vi "Autonics_1Scan_KAERI_lab2.vi"() -> ()   [LabVIEW 2018]
uses:
  <vilib>/Platform/NI_3dgraph.lvlib
  <vilib>/Utility/file.llb/Write To Spreadsheet File (DBL).vi
  <vilib>/Analysis/Matrix/Datatypes/RealMatrix.ctl
  <vilib>/Analysis/Matrix/NI_Matrix.lvlib
  <resource>/objmgr/daqmx.rc
  <vilib>/Instr/_visa.llb/VISA Configure Serial Port (Instr).vi
  <vilib>/DAQmx/configure/trigger.llb/DAQmx Start Trigger (Digital Edge).vi
  <vilib>/DAQmx/read.llb/DAQmx Read (Analog 2D DBL NChan NSamp).vi
  <vilib>/DAQmx/configure/timing.llb/DAQmx Timing (Sample Clock).vi
  <vilib>/DAQmx/create/channels.llb/DAQmx Create Channel (AI-Voltage-Basic).vi
  <vilib>/Analysis/NI_AALPro.lvlib
  <vilib>/Utility/file.llb/Read From Spreadsheet File (DBL).vi
  <vilib>/Analysis/2dsp.llb/Real FFT.vi
  <vilib>/Analysis/3filter.llb/Filter Passband Type.ctl
  <vilib>/Analysis/NI_AALBase.lvlib
panel:
  in  "Inverse":bool
  out "Sum Abs":dbl
  in  "Even":bool
  in  "Odd":bool
  in  "Scan Mode":bool
  in  "Save Analysis":bool caption="Save Process"
  in  "Open":bool
  in  "Filter?":bool
  in  "Direction":u16(ring) items=["X-dir", "Y-dir"]
  in  "filter type":T1
  in  "Sampling Hz":dbl=1000.0
  in  "High Cutoff Hz":dbl=300.0
  in  "Low Cutoff Hz":dbl=50.0
  in  "Order":dbl=2.0
  in  "Transpose ?":bool
  in  "3D Surface Analysis":refnum<k7>(container)
  in  "Color Min":dbl step=0.01
  in  "Color Max":dbl=1.0 step=0.01
  in  "Auto Scale ?":bool
  in  "Area View":bool
  out "Cursor X":dbl=1.0
  out "Cursor Y":dbl=1.0
  out "Cursor Z":dbl=1.0
  out "Section View Y":dbl[](graph) caption="Section View"
  in  "Line X":dbl
  in  "Line Y":dbl
  in  "Repair Line X":bool
  in  "Repair Line Y":bool
  in  "Back data Analysis":bool
  in  "dX":bool
  in  "dY":bool
  out "XY Graph":cluster{"Array Repaired":dbl[], dbl[]}(graph)
  in  "X-max":dbl
  in  "X-min":dbl
  in  "Trim Data":bool
  in  "Y-max":dbl
  in  "Y-min":dbl
  in  "ViewMode Analysis":i32(ring) items=["cwViewXYPlane", "cwViewXZPlane", "cwViewYZPlane", "cwViewUserDefined"]
  in  "Plot style Analysis":i32(ring)=5 items=["cwLine"=1, "cwPoint"=2, "cwLinePoint"=3, "cwHiddenLine"=4, "cwSurface"=5, "cwSurfaceLine"=6, "cwSurfaceNormal"=7, "cwContourLine"=8, "cwSurfaceContour"=9]
  out "Section View 2":dbl[](graph) caption="Section View"
  in  "Scan Distance":dbl=350.0
  in  "Multiplier":dbl=10.0
  in  "Save Button":bool caption="Save Process"
  in  "ViewMode":i32(ring) items=["cwViewXYPlane", "cwViewXZPlane", "cwViewYZPlane", "cwViewUserDefined"]
  in  "Back data":bool
  in  "Data Type":u16(ring) items=["Normal", "dX", "dY"]
  in  "Sampling Rate(Hz)":dbl=15000.0
  in  "Samples per Channels":i32=1000
  in  "Min Volts":dbl=-10.0 format="%0.2f"
  in  "Max Volts":dbl=10.0 format="%0.2f"
  in  "Channels":tag="Dev3/ai0:63"
  in  "Scan Step (mm)":dbl=1.0
  in  "Scan":bool
  in  "Plot style":i32(ring)=5 items=["cwLine"=1, "cwPoint"=2, "cwLinePoint"=3, "cwHiddenLine"=4, "cwSurface"=5, "cwSurfaceLine"=6, "cwSurfaceNormal"=7, "cwContourLine"=8, "cwSurfaceContour"=9]
  in  "3D Surface":refnum<k7>(container)
  in  "Flow control":u16(ring) items=["None", "XON/XOFF", "RTS/CTS", "XON/XOFF & RTS/CTS", "DTR/DSR", "XON/XOFF & DTR/DSR"]
  in  "Stop bits":u16(ring)=10 items=["1.0"=10, "1.5"=15, "2.0"=20]
  in  "Parity":dbl
  in  "Data bits":u16=8 min=5 max=8 step=1
  in  "Baud Rate":u32=57600
  in  "COM Port":refnum<visa-resource-name>="COM3"
  in  "Travel per Pulse (mm)":dbl=0.002
  in  "Speed (mm/s)":dbl=10.0
  out "Current  Position (mm)":dbl format="%#_4g"
  in  "Move Distance (mm)":dbl=20.0
  in  "Stop Scan":bool
  in  "Stop":bool
  in  "Home":bool
  in  "Right":bool
  in  "Left":bool
  # "SCANNER CONTROL"
  # "BOBBIN-TYPE MAGNETIC CAMERA"
  # "CHANNELS"
  # "COM Setting"
  # "TIMING"
  # "DATA ANALYSIS"
  # "Filters"
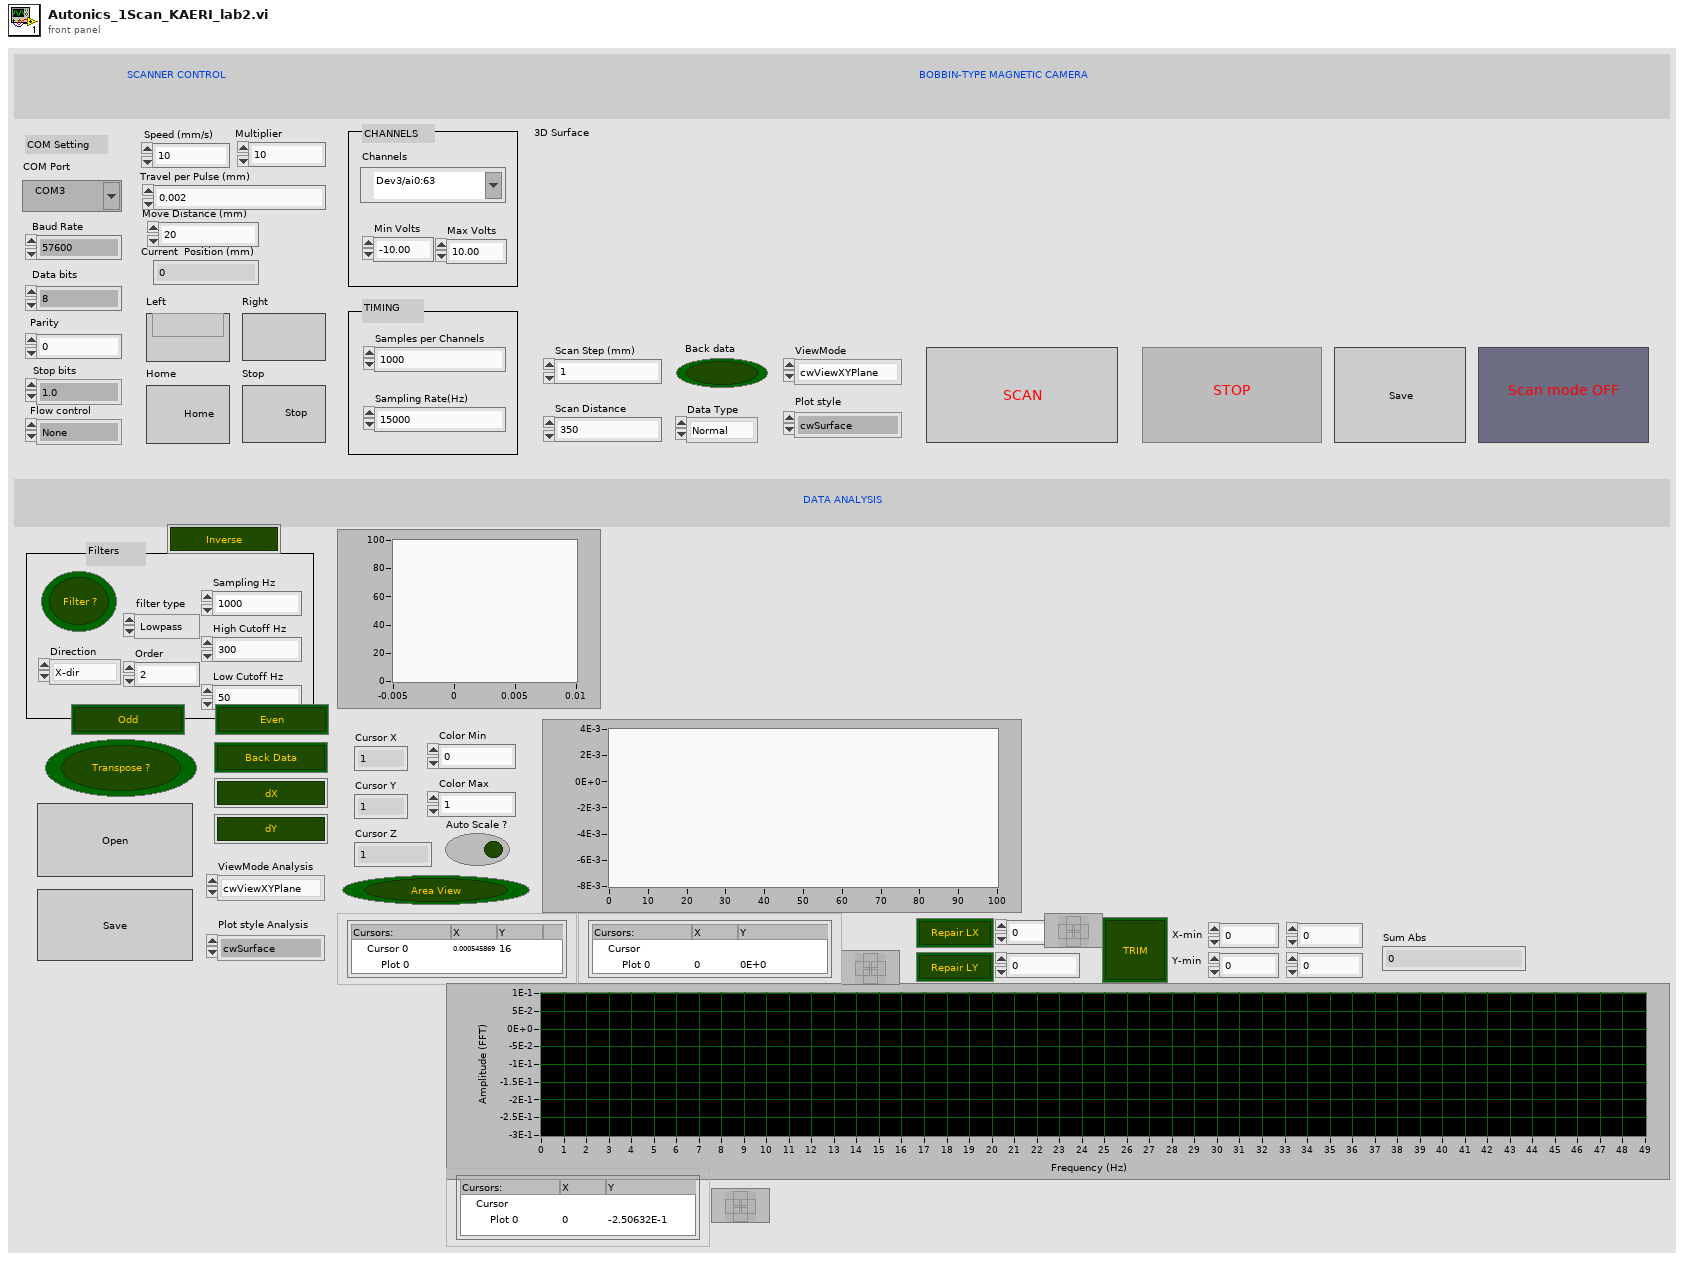
[diagram p1: front panel]
types:
  T1 = typedef "NI_AALBase.lvlib/Filter Passband Type.ctl" = enum32{"Lowpass", "Highpass", "Bandpass", "Bandstop"}
  T2 = typedef "NI_Matrix.lvlib/RealMatrix.ctl" = dbl[][]
  T3 = enum32{"Invalid", "Standard", "Closed", "Hidden", "Minimized", "Maximized"}
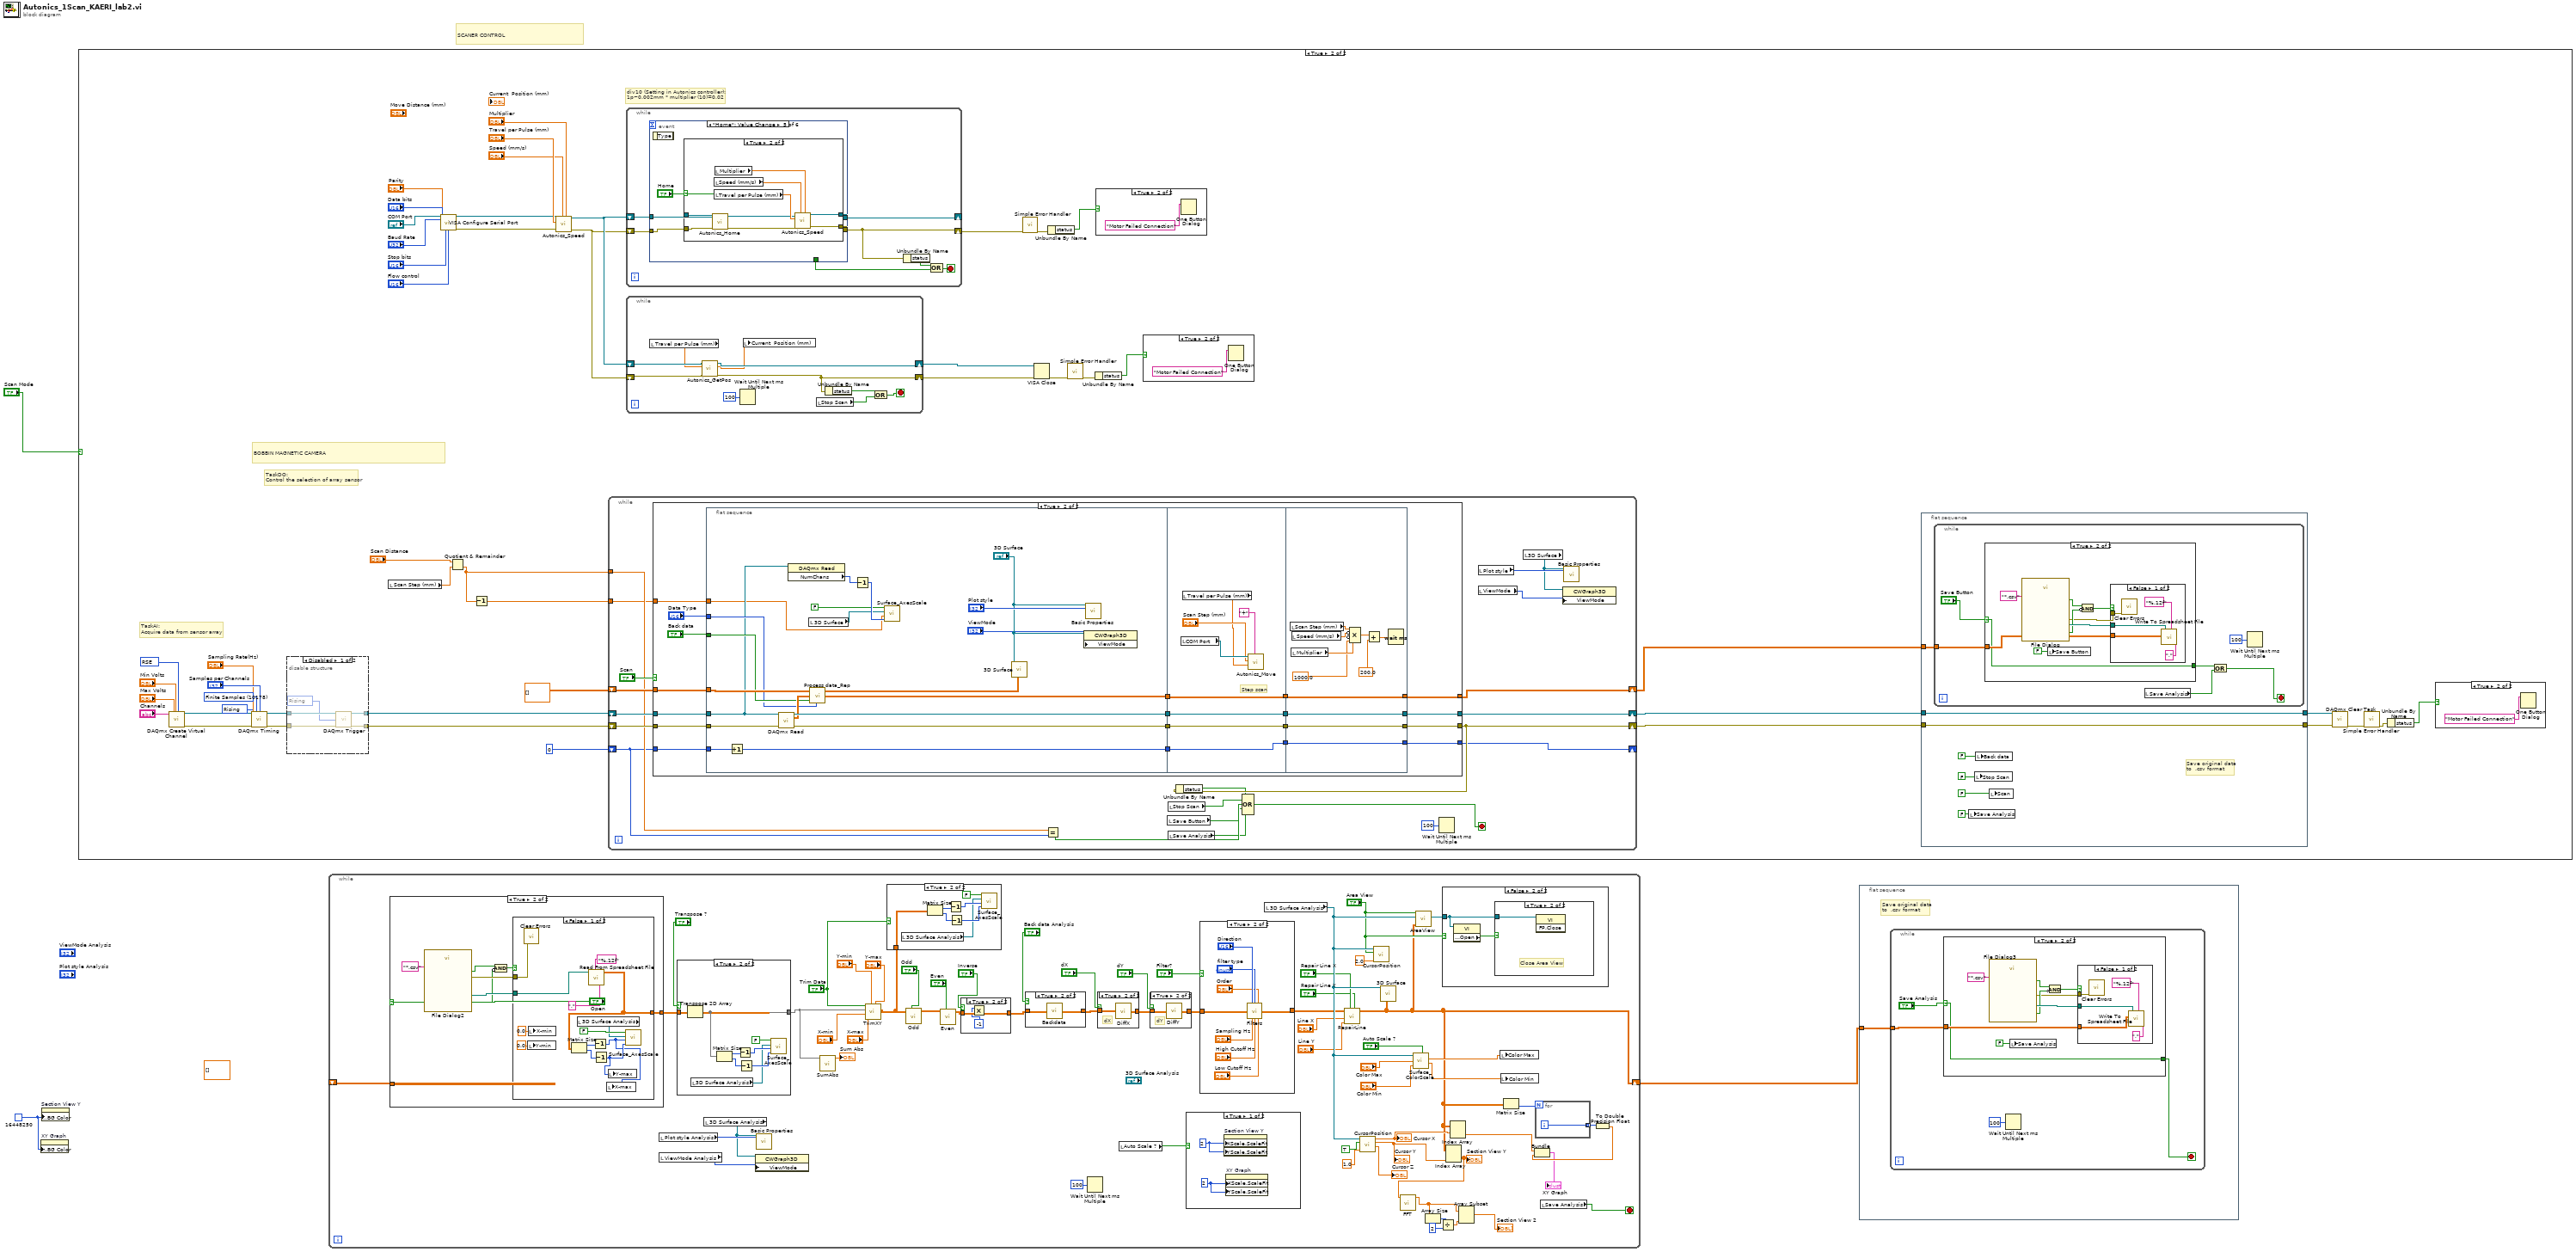
[diagram p0: block diagram]
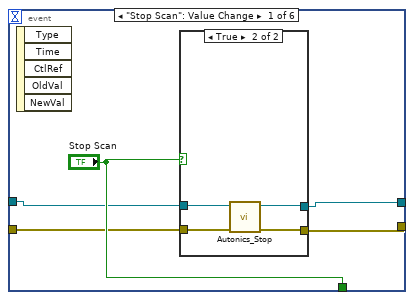
[diagram p5: hidden frame]
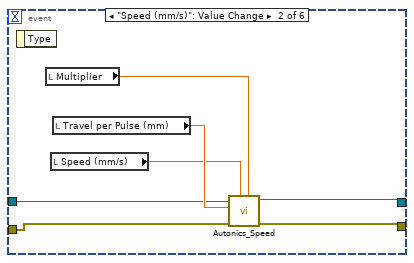
[diagram p7: hidden frame]
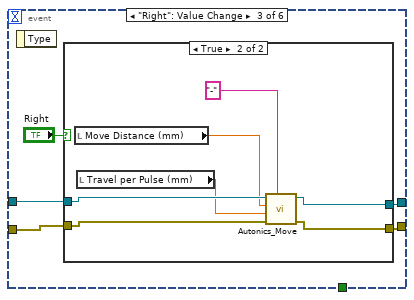
[diagram p8: hidden frame]
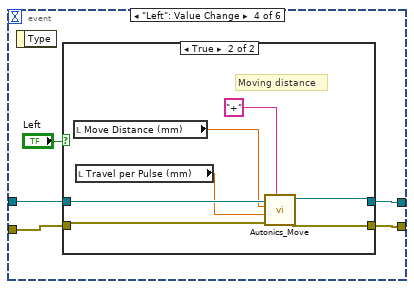
[diagram p10: hidden frame]
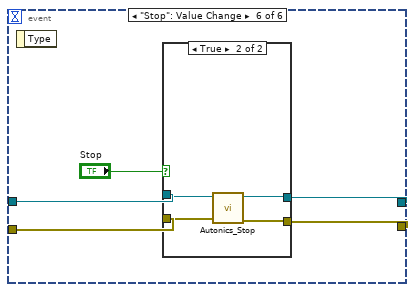
[diagram p13: hidden frame]
diagram:
  w2 = u32 16448250
  (unwired) T2 [] ("Output (Matrix)")
  # "SCANER CONTROL"
  n1 = property on="XY Graph" class="XYGraph (strict)"("Plot Area:Colors:BG Color"=w2) -> ()  [unwired: 2 in, 2 out]
  n2 = property on="Section View Y" class="WFGraph (strict)"("Plot Area:Colors:BG Color"=w2) -> ()  [unwired: 2 in, 2 out]
  n3 = case shown="True" "Scan Mode" {
    frame False {
    }
    frame True {
      w35 = 10280 items=["Rising"=10280, "Falling"=10171] ("active edge")
      w44 = 10083 items=["default"=-1, "RSE"=10083, "NRSE"=10078, "Differential"=10106, "Pseudodifferential"=12529] ("input terminal configuration")
      w45 = 10178 items=["Finite Samples"=10178, "Continuous Samples"=10123, "Hardware Timed Single Point"=12522] ("sample mode")
      # "div10 (Setting in Autonics controller):\n1p~0.002mm * multiplier (10)=0.02"
      # "TaskAI:\nAcquire data from sensor array"
      # "TaskDO: \nControl the selection of array sensor"
      # "BOBBIN MAGNETIC CAMERA"
      n4 = call-poly <vilib>:"DAQmx Create Virtual Channel.vi"("maximum value"="Max Volts", "minimum value"="Min Volts", "input terminal configuration"=w44, "physical channels"="Channels") -> ("task out"=w52:refnum<k21>, "error out"=w51:errorcluster)  [unwired: 10 in]
      n5 = call-poly <vilib>:"DAQmx Timing.vi"("task/channels in"=w52, "sample mode"=w45, "samples per channel"="Samples per Channels", "rate"="Sampling Rate(Hz)", "active edge"=w35, "error in"=w51) -> ("task out"=w34:refnum<k21>, "error out"=w33:errorcluster)  [unwired: 8 in]
      n6 = disable-structure shown="Disabled" {
        disable-tunnel: w34 -> [w151 w153]
        disable-tunnel: [w150 w153] -> w29
        disable-tunnel: w33 -> [w149 w152]
        disable-tunnel: [w148 w152] -> w32
        frame Disabled {
          w147 = 10280 items=["Rising"=10280, "Falling"=10171] ("edge")
          n7 = call-poly <vilib>:"DAQmx Trigger.vi"("task/channels in"=w151, "edge"=w147, "error in"=w149) -> ("task out"=w150:refnum<k21>, "source"=w146:tag, "error out"=w148:errorcluster)  [unwired: 10 in]
        }
        frame Enabled {
        }
      }
      n8 = local read "Scan Step (mm)"() -> (w43:dbl)
      n9 = call-poly "VISA Configure Serial Port"("VISA resource name"="COM Port", "baud rate (9600)"="Baud Rate", "data bits (8)"="Data bits", "parity (0:none)"="Parity", "stop bits (10: 1 bit)"="Stop bits", "flow control (0:none)"="Flow control") -> ("VISA resource name out"=w9:refnum<visa-resource-name>, "error out"=w8:errorcluster)  [unwired: 8 in]
      n10 = Quotient & Remainder(x="Scan Distance", y=w43) -> (floor(x/y)=w31:dbl)  [unwired: 1 out]
      n11 = Decrement(x=w31) -> (x-1=w27:dbl)
      n12 = call "Autonics_Speed.vi"("Multiplier"="Multiplier", "Speed (mm/s)"="Speed (mm/s)", "error in (no error)"=w8, "Travel per  Pulse"="Travel per Pulse (mm)", "VISA resource name"=w9) -> ("error out"=w13:errorcluster, "VISA resource name out"=w14:refnum<visa-resource-name>)  [unwired: 5 in]
      n13 = while {
        shift-right: [w185] -> w28
        shift-left: T2 [] ("Output (Matrix)") -> [w201]
        shift-right: [w199] -> w39
        shift-left: w29 -> [w200]
        shift-right: [w195] -> w37
        shift-left: w32 -> [w202]
        shift-right: [w193] -> _
        shift-left: 0 -> [w191]
        tunnel: w31 -> [w192]
        tunnel: w27 -> [w184]
        stop <- w198 stop-if-true
        n14 = case shown="True" "Scan" {
          tunnel: w200 -> [w205 w225]
          tunnel: w202 -> [w204 w224]
          tunnel: w201 -> [w203 w223]
          tunnel: [w205 w219] -> w199
          tunnel: [w204 w218] -> w195
          tunnel: [w203 w208] -> w185
          tunnel: [w206 w215] -> w193
          tunnel: w191 -> [w206 w213]
          tunnel: w184 -> [_ w207]
          frame False {
          }
          frame True {
            n15 = flat-sequence {
              tunnel: [w244] -> w222
              tunnel: [w235] -> w221
              tunnel: [w243] -> w220
              tunnel: [w234] -> w214
              tunnel: w225 -> [w227]
              tunnel: w224 -> [w245]
              tunnel: w223 -> [w239]
              tunnel: "Back data" -> [w237]
              tunnel: "Data Type" -> [w236]
              tunnel: w213 -> [w233]
              tunnel: w207 -> [w226]
              tunnel: w222 -> [w253]
              tunnel: w221 -> [w252]
              tunnel: w220 -> [w251]
              tunnel: w214 -> [w250]
              tunnel: [w253] -> w212
              tunnel: [w252] -> w211
              tunnel: [w251] -> w210
              tunnel: [w250] -> w209
              tunnel: [w261] -> w215
              tunnel: [w262] -> w218
              tunnel: [w263] -> w208
              tunnel: [w264] -> w219
              tunnel: w212 -> [w264]
              tunnel: w211 -> [w263]
              tunnel: w210 -> [w262]
              tunnel: w209 -> [w261]
              frame #0 {
                n16 = Increment(x=w233) -> (x+1=w234:i32)
                n17 = call-poly <vilib>:"DAQmx Read.vi"("task/channels in"=w227, "error in"=w245) -> ("task out"=w244:refnum<k21>, "data"=w238:dbl[][], "error out"=w243:errorcluster)  [unwired: 11 in]
                n18 = property class="DAQmx Read"(reference=w227) -> ("NumChans"=w230:u32)  [unwired: 1 in, 2 out]
                n19 = local read "3D Surface"() -> (w229:refnum<k7>)
                n20 = call "Process data_Rep.vi"("Initial Matrix"=w239, "Input Matrix"=w238, "Back Data"=w237, "Data Type"=w236) -> ("Process Output (Matrix)"=w232:T2, "Output (Matrix)"=w235:T2)  [unwired: 2 in]
                n21 = Decrement(x=w230) -> (x-1=w231:u32)
                n22 = call "Surface_AxesScale.vi"("Y-axis Max"=w231, "X-axis max"=w226, "3D Surface"=w229, "Auto Scale"=FALSE) -> ()  [unwired: 8 in]
                n23 = call <vilib>:"3D Surface.vi"("z matrix"=w232, "3D graph"="3D Surface") -> ()  [unwired: 8 in, 2 out]
                n24 = property class="CWGraph3D"(reference="3D Surface", "ViewMode"="ViewMode") -> ()  [unwired: 1 in, 2 out]
                n25 = call <vilib>:"Basic Properties.vi"("3D graph"="3D Surface", "plot style"="Plot style") -> ()  [unwired: 12 in, 2 out]
              }
              frame #1 {
                # "Step scan"
                n26 = local read "COM Port"() -> (w249:refnum<visa-resource-name>)
                n27 = local read "Travel per Pulse (mm)"() -> (w247:dbl)
                n28 = call "Autonics_Move.vi"("Direction (+)"="+", "Travel per Pulse (mm)"=w247, "Move Distance (mm)"="Scan Step (mm)", "VISA resource name"=w249) -> ()  [unwired: 6 in, 2 out]
              }
              frame #2 {
                n29 = local read "Scan Step (mm)"() -> (w256:dbl)
                n30 = local read "Multiplier"() -> (w255:dbl)
                n31 = local read "Speed (mm/s)"() -> (w257:dbl)
                n32 = Compound Arithmetic op=MULTIPLY(w256, invert w257, invert w255, 1000.0 ("value")) -> (w258:dbl)
                n33 = Add(x=w258, y=200.0) -> (x+y=w260:dbl)
                n34 = Wait (ms)(milliseconds to wait=w260) -> ()  [unwired: 1 out]
              }
            }
          }
        }
        n35 = Equal?(x=w192, y=w191) -> (x = y?=w190:bool)
        n36 = local read "Save Button"() -> (w183:bool)
        n37 = local read "Stop Scan"() -> (w196:bool)
        n38 = local read "Save Analysis"() -> (w182:bool)
        n39 = Unbundle By Name(w195) -> ("status"=w194:bool)
        n40 = Compound Arithmetic op=OR(w194, w196, w190, w183, w182) -> (w198:bool)
        n41 = Wait Until Next ms Multiple(millisecond multiple=u32 100) -> ()  [unwired: 1 out]
        n42 = local read "Plot style"() -> (w188:i32)
        n43 = local read "ViewMode"() -> (w187:i32)
        n44 = local read "3D Surface"() -> (w186:refnum<k7>)
        n45 = property class="CWGraph3D"(reference=w186, "ViewMode"=w187) -> ()  [unwired: 1 in, 2 out]
        n46 = call <vilib>:"Basic Properties.vi"("3D graph"=w186, "plot style"=w188) -> ()  [unwired: 12 in, 2 out]
      }
      n47 = while {
        shift-right: [w71] -> _
        shift-left: w14 -> [w70]
        shift-right: [w67] -> w17
        shift-left: w13 -> [w69]
        stop <- w66 stop-if-true
        n48 = event shown="[4] \"Home\": Value Change" {
          selector: _ -> [_ _ _ _ _ _]
          dyn-events: _ -> [_ _ _ _ _ _]
          timeout: _ -> [_ _ _ _ _ _]
          tunnel: w70 -> [w75 w88 w92 w106 w122 w136]
          tunnel: w69 -> [w74 w87 w91 w105 w121 w135]
          tunnel: [w73 w83 w94 w108 w119 w138] -> w71
          tunnel: [w72 w84 w93 w107 w118 w137] -> w67
          tunnel: ["Stop Scan" _ _ _ _ _] -> w65
          event "Stop Scan": Value Change {
            n49 = event-data() -> ()  [unwired: 1 in, 5 out]
            n50 = case shown="True" "Stop Scan" {
              tunnel: [w78 w81] -> w73
              tunnel: [w77 w82] -> w72
              tunnel: w75 -> [w78 w80]
              tunnel: w74 -> [w77 w79]
              frame False {
              }
              frame True {
                n51 = call "Autonics_Stop.vi"("error in (no error)"=w79, "VISA resource name"=w80) -> ("error out"=w82:errorcluster, "VISA resource name out"=w81:refnum<visa-resource-name>)  [unwired: 8 in]
              }
            }
          }
          event "Speed (mm/s)": Value Change {
            n52 = event-data() -> ()  [unwired: 1 in, 1 out]
            n53 = local read "Multiplier"() -> (w85:dbl)
            n54 = local read "Speed (mm/s)"() -> (w86:dbl)
            n55 = local read "Travel per Pulse (mm)"() -> (w89:dbl)
            n56 = call "Autonics_Speed.vi"("Multiplier"=w85, "Speed (mm/s)"=w86, "error in (no error)"=w87, "Travel per  Pulse"=w89, "VISA resource name"=w88) -> ("error out"=w84:errorcluster, "VISA resource name out"=w83:refnum<visa-resource-name>)  [unwired: 5 in]
          }
          event "Right": Value Change {
            n57 = event-data() -> ()  [unwired: 1 in, 1 out]
            n58 = case shown="True" "Right" {
              tunnel: [w95 w101] -> w94
              tunnel: [w96 w100] -> w93
              tunnel: w92 -> [w95 w103]
              tunnel: w91 -> [w96 w102]
              frame False {
              }
              frame True {
                n59 = local read "Move Distance (mm)"() -> (w99:dbl)
                n60 = local read "Travel per Pulse (mm)"() -> (w98:dbl)
                n61 = call "Autonics_Move.vi"("Direction (+)"="-", "error in (no error)"=w102, "Travel per Pulse (mm)"=w98, "Move Distance (mm)"=w99, "VISA resource name"=w103) -> ("error out"=w100:errorcluster, "VISA resource name out"=w101:refnum<visa-resource-name>)  [unwired: 5 in]
              }
            }
          }
          event "Left": Value Change {
            n62 = event-data() -> ()  [unwired: 1 in, 1 out]
            n63 = case shown="True" "Left" {
              tunnel: [w110 w115] -> w108
              tunnel: [w109 w114] -> w107
              tunnel: w106 -> [w110 w117]
              tunnel: w105 -> [w109 w116]
              frame False {
              }
              frame True {
                # "Moving distance"
                n64 = local read "Move Distance (mm)"() -> (w112:dbl)
                n65 = local read "Travel per Pulse (mm)"() -> (w111:dbl)
                n66 = call "Autonics_Move.vi"("Direction (+)"="+", "error in (no error)"=w116, "Travel per Pulse (mm)"=w111, "Move Distance (mm)"=w112, "VISA resource name"=w117) -> ("error out"=w114:errorcluster, "VISA resource name out"=w115:refnum<visa-resource-name>)  [unwired: 5 in]
              }
            }
          }
          event "Home": Value Change {
            n67 = event-data() -> ()  [unwired: 1 in, 1 out]
            n68 = case shown="True" "Home" {
              tunnel: [w124 w126] -> w119
              tunnel: [w123 w125] -> w118
              tunnel: w122 -> [w124 w133]
              tunnel: w121 -> [w123 w132]
              frame False {
              }
              frame True {
                n69 = call "Autonics_Home.vi"("error in (no error)"=w132, "VISA resource name"=w133) -> ("error out"=w127:errorcluster, "VISA resource name out"=w128:refnum<visa-resource-name>)  [unwired: 8 in]
                n70 = local read "Speed (mm/s)"() -> (w130:dbl)
                n71 = local read "Travel per Pulse (mm)"() -> (w131:dbl)
                n72 = local read "Multiplier"() -> (w129:dbl)
                n73 = call "Autonics_Speed.vi"("Multiplier"=w129, "Speed (mm/s)"=w130, "error in (no error)"=w127, "Travel per  Pulse"=w131, "VISA resource name"=w128) -> ("error out"=w125:errorcluster, "VISA resource name out"=w126:refnum<visa-resource-name>)  [unwired: 5 in]
              }
            }
          }
          event "Stop": Value Change {
            n74 = event-data() -> ()  [unwired: 1 in, 1 out]
            n75 = case shown="True" "Stop" {
              tunnel: [w140 w141] -> w138
              tunnel: [w139 w144] -> w137
              tunnel: w136 -> [w140 w143]
              tunnel: w135 -> [w139 w142]
              frame False {
              }
              frame True {
                n76 = call "Autonics_Stop.vi"("error in (no error)"=w142, "VISA resource name"=w143) -> ("error out"=w144:errorcluster, "VISA resource name out"=w141:refnum<visa-resource-name>)  [unwired: 8 in]
              }
            }
          }
        }
        n77 = Unbundle By Name(w67) -> ("status"=w68:bool)
        n78 = Compound Arithmetic op=OR(w68, w65) -> (w66:bool)
      }
      n79 = while {
        shift-right: [w58] -> w16
        shift-left: w14 -> [w60]
        shift-right: [w57] -> w15
        shift-left: w13 -> [w59]
        stop <- w61 stop-if-true
        n80 = local read "Travel per Pulse (mm)"() -> (w56:dbl)
        n81 = call "Autonics_GetPos.vi"("error in (no error)"=w59, "Travel per Pulse (mm)"=w56, "VISA resource name"=w60) -> ("error out"=w57:errorcluster, "Current  Position (mm)"=w55:dbl, "VISA resource name out"=w58:refnum<visa-resource-name>)  [unwired: 6 in]
        n82 = Wait Until Next ms Multiple(millisecond multiple=u32 100) -> ()  [unwired: 1 out]
        n83 = local write "Current  Position (mm)"(w55) -> ()
        n84 = local read "Stop Scan"() -> (w62:bool)
        n85 = Unbundle By Name(w57) -> ("status"=w63:bool)
        n86 = Compound Arithmetic op=OR(w63, w62) -> (w61:bool)
      }
      n87 = call <vilib>:"Simple Error Handler.vi"("error in (no error)"=w17) -> ("error out"=w6:errorcluster)  [unwired: 4 in, 4 out]
      n88 = VISA Close(VISA resource name=w16, error in (no error)=w15) -> (error out=w20:errorcluster)
      n89 = Unbundle By Name(w6) -> ("status"=w7:bool)
      n90 = call <vilib>:"Simple Error Handler.vi"("error in (no error)"=w20) -> ("error out"=w4:errorcluster)  [unwired: 4 in, 4 out]
      n91 = Unbundle By Name(w4) -> ("status"=w5:bool)
      n92 = case shown="True" w7 {
        frame False {
        }
        frame True {
          n93 = One Button Dialog(message="Motor Failed Connection") -> ()  [unwired: 1 in, 1 out]
        }
      }
      n94 = case shown="True" w5 {
        frame False {
        }
        frame True {
          n95 = One Button Dialog(message="Motor Failed Connection") -> ()  [unwired: 1 in, 1 out]
        }
      }
      n96 = flat-sequence {
        tunnel: w39 -> [w160]
        tunnel: [w160] -> w38
        tunnel: w37 -> [w159]
        tunnel: [w159] -> w36
        tunnel: w28 -> [w155]
        frame #0 {
          # "Save original data\nto  .csv format"
          n97 = while {
            tunnel: w155 -> [w166]
            stop <- w161 stop-if-true
            n98 = case shown="True" "Save Button" {
              selector: "Save Button" -> [w167 w169]
              tunnel: w166 -> [_ w176]
              tunnel: [w167 w169] -> w163
              frame False {
              }
              frame True {
                n99 = call "File Dialog"("pattern (all files)"="*.csv") -> ("selected path"=w174:path, "exists"=w172:bool, "cancelled"=w173:bool, "error out"=w170:errorcluster)  [unwired: 11 in]
                n100 = local write "Save Button"(FALSE ("Save Button")) -> ()
                n101 = Compound Arithmetic op=AND(w173, invert w172) -> (w171:bool)
                n102 = case shown="False" w171 {
                  tunnel: w176 -> [w181 _]
                  tunnel: w174 -> [w179 _]
                  tunnel: w170 -> [w177 _]
                  frame False {
                    n103 = call <vilib>:"Clear Errors.vi"("error in (no error)"=w177) -> ()  [unwired: 5 in, 2 out]
                    n104 = call-poly <vilib>:"Write To Spreadsheet File.vi"("delimiter (\\t)"="," ("delimiter (\\t)"), "format (%.3f)"="%.12f", "2D data"=w181, "file path (dialog if empty)"=w179) -> ()  [unwired: 4 in, 1 out]
                  }
                  frame True {
                  }
                }
              }
            }
            n105 = local read "Save Analysis"() -> (w162:bool)
            n106 = Compound Arithmetic op=OR(w163, w162) -> (w161:bool)
            n107 = Wait Until Next ms Multiple(millisecond multiple=u32 100) -> ()  [unwired: 1 out]
          }
          n108 = local write "Save Analysis"(FALSE ("Tranpose ?")) -> ()
          n109 = local write "Stop Scan"(FALSE ("Exit")) -> ()
          n110 = local write "Back data"(FALSE ("Back data")) -> ()
          n111 = local write "Scan"(FALSE ("Scan")) -> ()
        }
      }
      n112 = call <vilib>:"DAQmx Clear Task.vi"("task in"=w38, "error in"=w36) -> ("error out"=w40:errorcluster)  [unwired: 13 in]
      n113 = call <vilib>:"Simple Error Handler.vi"("error in (no error)"=w40) -> ("error out"=w25:errorcluster)  [unwired: 4 in, 4 out]
      n114 = Unbundle By Name(w25) -> ("status"=w26:bool)
      n115 = case shown="True" w26 {
        frame False {
        }
        frame True {
          n116 = One Button Dialog(message="Motor Failed Connection") -> ()  [unwired: 1 in, 1 out]
        }
      }
    }
  }
  n117 = while {
    shift-right: [w291] -> w3
    shift-left: _ -> [w326]
    stop <- w321 stop-if-true
    n118 = case shown="True" "Open" {
      tunnel: w326 -> [w355 _]
      tunnel: [w355 w362] -> w317
      frame False {
      }
      frame True {
        n119 = call "File Dialog2"("pattern (all files)"="*.csv") -> ("selected path"=w361:path, "exists"=w356:bool, "cancelled"=w357:bool, "error out"=w359:errorcluster)  [unwired: 11 in]
        n120 = Compound Arithmetic op=AND(w357, invert w356) -> (w358:bool)
        n121 = case shown="False" w358 {
          tunnel: w361 -> [w375 _]
          tunnel: [w374 _] -> w362
          tunnel: w359 -> [w373 _]
          frame False {
            n122 = call <vilib>:"Clear Errors.vi"("error in (no error)"=w373) -> ()  [unwired: 5 in, 2 out]
            n123 = local write "Y-min"(0.0 ("Y-min")) -> ()
            n124 = local write "X-min"(0.0 ("X-min")) -> ()
            n125 = local read "3D Surface Analysis"() -> (w367:refnum<k7>)
            n126 = call-poly <vilib>:"Read From Spreadsheet File.vi"("delimiter (\\t)"="," ("delimiter (\\t)"), "format (%.3f)"="%.12f", "file path (dialog if empty)"=w375) -> ("all rows"=w374:dbl[][])  [unwired: 4 in, 4 out]
            n127 = Matrix Size(0:w374) -> (1:w370:i32, 2:w369:i32)
            n128 = Decrement(x=w370) -> (x-1=w363:i32)
            n129 = Decrement(x=w369) -> (x-1=w364:i32)
            n130 = local write "X-max"(w363) -> ()
            n131 = local write "Y-max"(w364) -> ()
            n132 = call "Surface_AxesScale.vi"("Y-axis Max"=w364, "X-axis max"=w363, "3D Surface"=w367, "Auto Scale"=FALSE) -> ()  [unwired: 8 in]
          }
          frame True {
          }
        }
      }
    }
    n133 = local read "Plot style Analysis"() -> (w320:i32)
    n134 = local read "ViewMode Analysis"() -> (w319:i32)
    n135 = case shown="True" "Transpose ?" {
      tunnel: w317 -> [w376 w384]
      tunnel: [w376 w378] -> w269
      frame False {
      }
      frame True {
        n136 = Transpose 2D Array(2D array=w384) -> (transposed array=w378:dbl[][])
        n137 = local read "3D Surface Analysis"() -> (w377:refnum<k7>)
        n138 = Matrix Size(0:w378) -> (1:w379:i32, 2:w380:i32)
        n139 = Decrement(x=w379) -> (x-1=w382:i32)
        n140 = Decrement(x=w380) -> (x-1=w383:i32)
        n141 = call "Surface_AxesScale.vi"("Y-axis Max"=w383, "X-axis max"=w382, "3D Surface"=w377, "Auto Scale"=FALSE) -> ()  [unwired: 8 in]
      }
    }
    n142 = local read "3D Surface Analysis"() -> (w318:refnum<k7>)
    n143 = property class="CWGraph3D"(reference=w318, "ViewMode"=w319) -> ()  [unwired: 1 in, 2 out]
    n144 = call <vilib>:"Basic Properties.vi"("3D graph"=w318, "plot style"=w320) -> ()  [unwired: 12 in, 2 out]
    n145 = call "SumAbs.vi"("Array In"=w269) -> ("sum"=→"Sum Abs":dbl)  [unwired: 10 in]
    n146 = call "TrimXY.vi"("X-max"="Y-max", "X-min"="Y-min", "Y-max"="X-max", "Y-min"="X-min", "Array In"=w269, "Trim data"="Trim Data") -> ("Array Trim Out"=w273:dbl[][])  [unwired: 5 in]
    n147 = case shown="True" "Trim Data" {
      tunnel: w273 -> [_ w331]
      frame False {
      }
      frame True {
        n148 = local read "3D Surface Analysis"() -> (w332:refnum<k7>)
        n149 = Matrix Size(0:w331) -> (1:w333:i32, 2:w334:i32)
        n150 = Decrement(x=w333) -> (x-1=w336:i32)
        n151 = Decrement(x=w334) -> (x-1=w337:i32)
        n152 = call "Surface_AxesScale.vi"("Y-axis Max"=w337, "X-axis max"=w336, "3D Surface"=w332, "Auto Scale"=FALSE) -> ()  [unwired: 8 in]
      }
    }
    n153 = call "Odd.vi"("Odd"="Odd", "Array In"=w273) -> ("Array Out"=w271:dbl[][])  [unwired: 9 in]
    n154 = call "Even.vi"("Even"="Even", "Array In"=w271) -> ("Array Out"=w265:dbl[][])  [unwired: 9 in]
    n155 = case shown="True" "Inverse" {
      tunnel: [w327 w329] -> w266
      tunnel: w265 -> [w327 w330]
      frame False {
      }
      frame True {
        n156 = Multiply(x=-1, y=w330) -> (x*y=w329:dbl[][])
      }
    }
    n157 = case shown="True" "Back data Analysis" {
      tunnel: w266 -> [w394 w395]
      tunnel: [w394 w396] -> w302
      frame False {
      }
      frame True {
        n158 = call "Backdata.vi"("Input Matrix"=w395) -> ("Backdata (matrix)"=w396:T2)
      }
    }
    n159 = Wait Until Next ms Multiple(millisecond multiple=u32 100) -> ()  [unwired: 1 out]
    n160 = case shown="True" "dX" {
      tunnel: [w346 w348] -> w300
      tunnel: w302 -> [w346 w347]
      frame False {
      }
      frame True {
        # "dX"
        n161 = call "DiffX.vi"("Input Matrix"=w347) -> ("Diff X (Matrix)"=w348:T2)
      }
    }
    n162 = local read "Auto Scale ?"() -> (w281:bool)
    n163 = case shown="True" "dY" {
      tunnel: w300 -> [w343 w344]
      tunnel: [w343 w345] -> w298
      frame False {
      }
      frame True {
        # "dY"
        n164 = call "DiffY.vi"("Input Matrix"=w344) -> ("Diff Y (Matrix)"=w345:T2)
      }
    }
    n165 = case shown="True" w281 {
      frame True {
        w338 = u8 2 ("X Scale.Scale Fit")
        w339 = u8 2 ("X Scale.Scale Fit")
        n166 = property on="Section View Y" class="WFGraph (strict)"("XScale.ScaleFit"=w339, "YScale.ScaleFit"=w339) -> ()  [unwired: 2 in, 2 out]
        n167 = property on="XY Graph" class="XYGraph (strict)"("XScale.ScaleFit"=w338, "YScale.ScaleFit"=w338) -> ()  [unwired: 2 in, 2 out]
      }
      frame False {
        w340 = u8 0 ("X Scale.Scale Fit")
        w341 = u8 0 ("X Scale.Scale Fit")
        n168 = property on="XY Graph" class="XYGraph (strict)"("XScale.ScaleFit"=w340, "YScale.ScaleFit"=w340) -> ()  [unwired: 2 in, 2 out]
        n169 = property on="Section View Y" class="WFGraph (strict)"("XScale.ScaleFit"=w341, "YScale.ScaleFit"=w341) -> ()  [unwired: 2 in, 2 out]
      }
    }
    n170 = case shown="True" "Filter?" {
      tunnel: [w385 w387] -> w297
      tunnel: w298 -> [w385 w386]
      frame False {
      }
      frame True {
        n171 = call "Filters.vi"("Direction"="Direction", "filter type"="filter type", "Order"="Order", "Input data"=w386, "Sampling Freq"="Sampling Hz", "High Cutoff Freq"="High Cutoff Hz", "Low Cutoff Freq"="Low Cutoff Hz") -> ("Filterd Data Matrix"=w387:T2)  [unwired: 8 in]
      }
    }
    n172 = local read "3D Surface Analysis"() -> (w316:refnum<k7>)
    n173 = call "RepairLine.vi"("Repair Line Col"="Repair Line Y", "Repair Line Row"="Repair Line X", "Line Col"="Line Y", "Line Row"="Line X", "Array In"=w297) -> ("Array Repaired"=w291:dbl[][])  [unwired: 6 in]
    n174 = call "CursorPosition.vi"("Cursor No."=1.0, "Cursor"=TRUE ("Visible"), "3D Surface Analysis"=w316) -> ("Cursor Z"=→"Cursor Z":dbl, "Cursor Y"=w307:dbl, "Cursor X"=w292:dbl)  [unwired: 6 in]
    "Cursor X" <- w292
    "Cursor Y" <- w307
    n175 = call "CursorPosition.vi"("Cursor No."=2.0, "Cursor"="Area View", "3D Surface Analysis"=w316) -> ()  [unwired: 6 in, 3 out]
    n176 = call <vilib>:"3D Surface.vi"("z matrix"=w291, "3D graph"=w316) -> ()  [unwired: 8 in, 2 out]
    n177 = call "Surface_ColorScale.vi"("ColorMapAutoScale"="Auto Scale ?", "Min"="Color Min", "Max"="Color Max", "3D Surface_"=w316) -> ("Min 2"=w311:dbl, "Max 2"=w312:dbl)  [unwired: 1 in, 2 out]
    n178 = call "AreaView.vi"("Real Matrix"=w291, "3D Surface Analysis"=w316, "Area View"="Area View") -> ("This VI"=w309:refnum<vi>)  [unwired: 7 in, 1 out]
    n179 = case shown="False" "Area View" {
      tunnel: w309 -> [w351 w353]
      frame True {
        # "Open Area View"
        n180 = invoke class="VI" method="FP.Open"(reference=w351, "Activate"=TRUE ("Activate?"), "State"=T3."Standard") -> ()  [unwired: 2 in, 5 out]
      }
      frame False {
        n181 = property class="VI"(reference=w353) -> ("Front Panel.Open"=w352:bool)  [unwired: 1 in, 2 out]
        n182 = case shown="True" w352 {
          tunnel: w353 -> [_ w354]
          frame False {
          }
          frame True {
            # "Close Area View"
            n183 = invoke class="VI" method="FP.Close"(reference=w354) -> ()  [unwired: 2 in, 3 out]
          }
        }
      }
    }
    n184 = Index Array(array=w291, index (col)=w307) -> (element=w274:dbl[])  [unwired: 1 in]
    "Section View Y" <- w274
    n185 = call-poly <vilib>:"FFT.vi"("X"=w274) -> ("FFT {X}"=w276:cdb[])  [unwired: 9 in, 1 out]
    n186 = Array Size(array=w276) -> (size(s)=w279:i32)
    n187 = Divide(x=w279, y=2) -> (x/y=w278:dbl)
    n188 = Index Array(array=w291, index (row)=w292) -> (element=w289:dbl[])  [unwired: 1 in]
    n189 = Array Subset(array=w276, length=w278) -> (→"Section View 2":cdb[])  [unwired: 1 in]
    n190 = local write "Color Max"(w312) -> ()
    n191 = local write "Color Min"(w311) -> ()
    n192 = Matrix Size(0:w291) -> (2:w290:i32)  [unwired: 1 out]
    n193 = for {
      N: w290 -> [_]
      tunnel: [w342] -> w288 mode=indexing
      i -> [w342]
    }
    n194 = local read "Save Analysis"() -> (w321:bool)
    n195 = To Double Precision Float(number=w288) -> (double precision float=w287:dbl[])
    n196 = Bundle("Array Repaired"=w289, w287) -> (→"XY Graph":cluster{"Array Repaired":dbl[], dbl[]})  [unwired: 1 in]
  }
  n197 = flat-sequence {
    tunnel: w3 -> [w397]
    frame #0 {
      # "Save original data\nto  .csv format"
      n198 = while {
        tunnel: w397 -> [w401]
        stop <- w399 stop-if-true
        n199 = case shown="True" "Save Analysis" {
          selector: "Save Analysis" -> [w402 w404]
          tunnel: w401 -> [_ w405]
          tunnel: [w402 w404] -> w399
          frame False {
          }
          frame True {
            n200 = call "File Dialog3"("pattern (all files)"="*.csv") -> ("selected path"=w410:path, "exists"=w408:bool, "cancelled"=w409:bool, "error out"=w406:errorcluster)  [unwired: 11 in]
            n201 = local write "Save Analysis"(FALSE ("Save Analysis")) -> ()
            n202 = Compound Arithmetic op=AND(w409, invert w408) -> (w407:bool)
            n203 = case shown="False" w407 {
              tunnel: w410 -> [w415 _]
              tunnel: w406 -> [w413 _]
              tunnel: w405 -> [w412 _]
              frame False {
                n204 = call <vilib>:"Clear Errors.vi"("error in (no error)"=w413) -> ()  [unwired: 5 in, 2 out]
                n205 = call-poly <vilib>:"Write To Spreadsheet File.vi"("delimiter (\\t)"="," ("delimiter (\\t)"), "format (%.3f)"="%.12f", "2D data"=w412, "file path (dialog if empty)"=w415) -> ()  [unwired: 4 in, 1 out]
              }
              frame True {
              }
            }
          }
        }
        n206 = Wait Until Next ms Multiple(millisecond multiple=u32 100) -> ()  [unwired: 1 out]
      }
    }
  }
